vi "QueueMultiPakect_Snapshot.vi"(8 "no error":errorcluster, 11 "EndSession":bool=TRUE) -> (0 "error out":errorcluster={"status"=FALSE, "code"=1073676294, "source"="VISA Read in SerialCOM.vi->Queue MultiPakect-13.vi->getvideo.vi->Focus Routine.vi->Focus Routine.vi.ProxyCaller"}, 1 "success?":bool=TRUE, 2 "ImageData":u8[](array[numeric]) format="%x", 5 "RecvBuff":string, 6 "Done":bool=TRUE)   [LabVIEW 2014]
doc: "Demonstrates general use of Obtain Queue, queues and the effects different settings have on queue behavior. It uses a queue to pass data between an Enqueue loop (producing data) and a Dequeue loop (consuming data). If both loops run at the same speed, the queue does not fill up.\n\nWhen the Enqueue loop runs fast and the Dequeue loop runs slow, the queue quickly fills up and the Enqueue loop must wait for the Dequeue loop to remove elements. If the Enqueue loop runs slow and the Dequeue loop runs fast, the queue is quickly emptied and the Dequeue loop must wait for the Enqueue loop to insert elements."
panel:
  out "SendEndSession":bool
  out "max":u32
  out "Raw Data":u8[](array[numeric]) format="%x"
  out "Num_images":dbl=2.0
  out "readtime 2":u32=395
  out "RecvBuff 2":string
  out "#Ends":u32
  out "source":string="VISA Read in SerialCOM.vi->Queue MultiPakect-13.vi->getvideo.vi->Focus Routine.vi->Focus Routine.vi.ProxyCaller"
  out "Pakect":u8[](array[numeric])=[152, 180, 0, 0, 18, 18, 18, 18, 19, 18, 19, 18, 18, 19, 18, 19, 18, 18, 18, 18, 18, 19, 18, 18, 18, 18, 18, 18, 18, 18, 18, 18, 18, 18, 19, 18, 19, 18, 18, 18, 18, 18, 19, 18, 18, 18, 18, 18, 18, 18, 18, 18, 19, 19, 18, 18, 18, 18, 19, 19, 18, 19, 18, 18, 18, 18, 18, 18, 18, 18, 18, 18, 19, 18, 19, 18, 19, 18, 19, 18, 18, 18, 18, 19, 18, 19, 18, 18, 18, 19, 19, 18, 18, 18, 18, 18, 18, 18, 18, 18, 18, 19, 18, 18, 18, 18, 18, 18, 19, 18, 18, 18, 19, 18, 18, 18, 19, 19, 18, 18, 18, 18, 19, 19, 18, 18, 18, 19, 19, 18, 18, 18, 18, 19, 18, 18, 18, 18, 18, 18, 18, 18, 18, 19, 18, 18, 18, 19, 18, 18, 18, 18, 244, 43]
  out "End paks":bool=TRUE
  out "Index":u32=200346
  out "#Pakects":u32=783
  out "# in queue":i32
  out "readtime":u32=395
  out "DeEnque Loop":i32=879
  out "StartTime":u32=22222026
  out "Bytes At Port Loop":i32=1757
  out "Bytes at Port":u32
  out "Enque Loop":i32=391
  out "Bytes Read":u32=200346
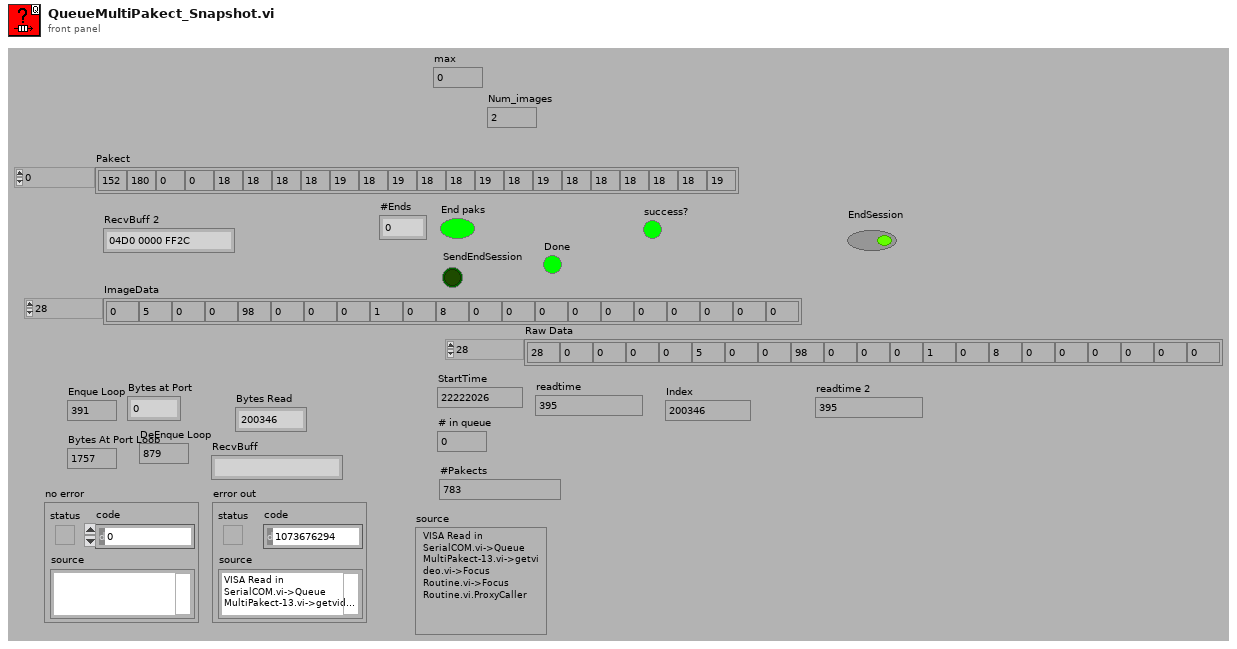
[diagram p1: front panel]
types:
  T1 = enum16{"OpenPort", "Initial Serial Port", "Write", "ByteRead", "Read", "ClearBuff", "Close"}
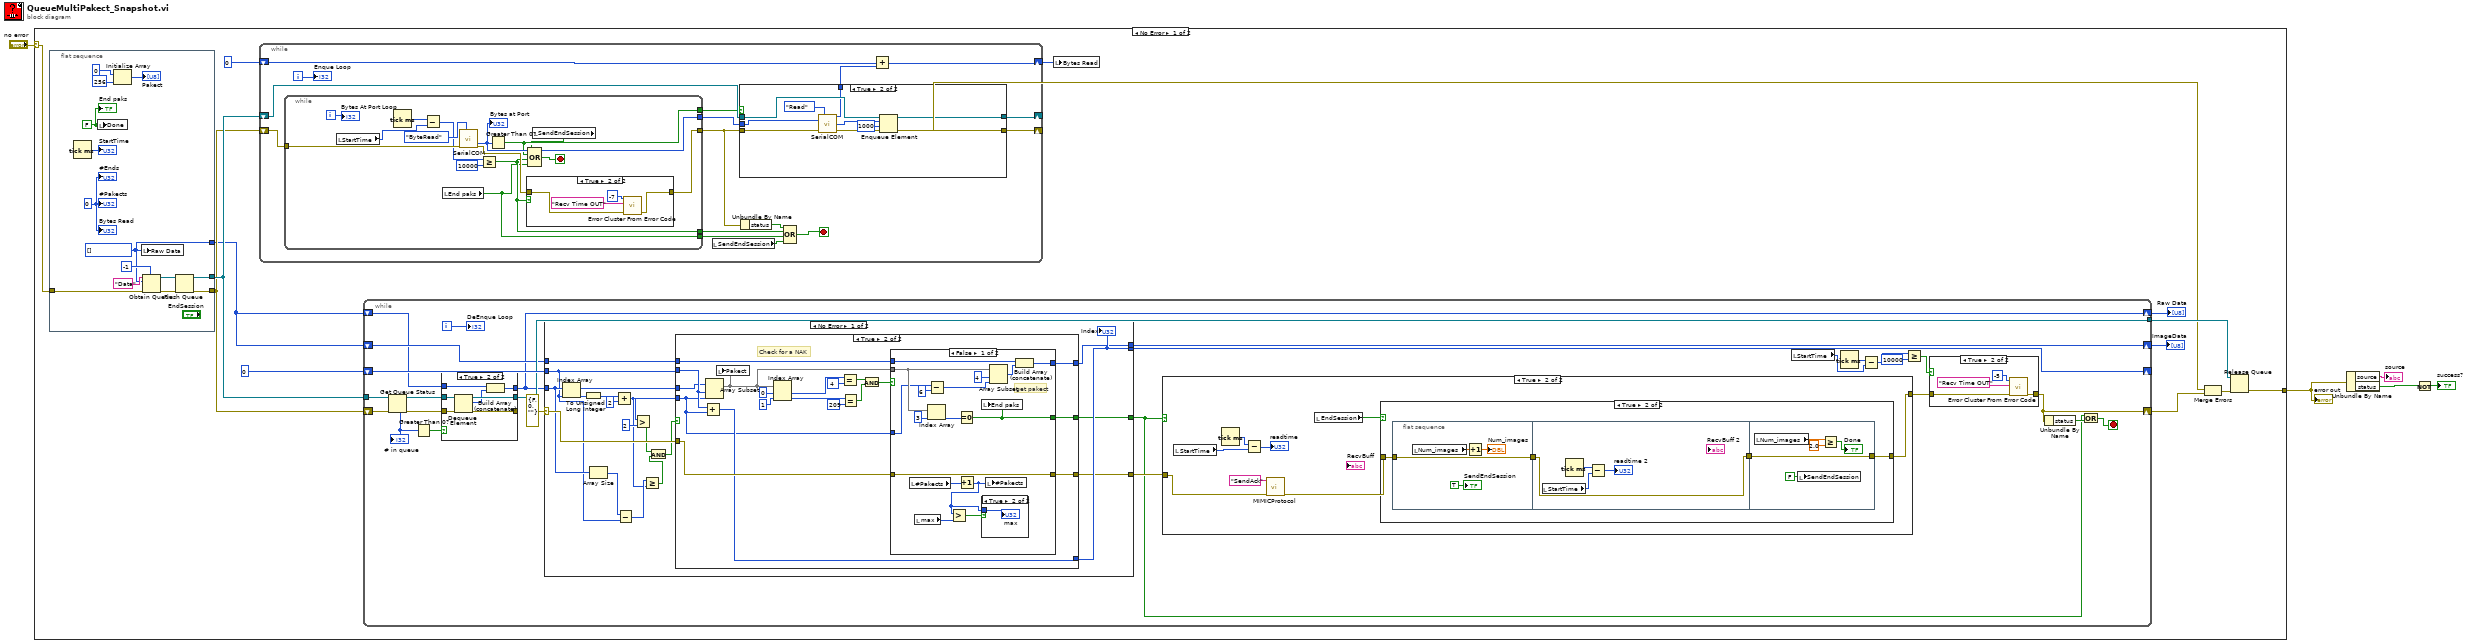
[diagram p0: block diagram]
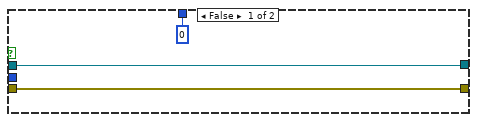
[diagram p3: hidden frame]
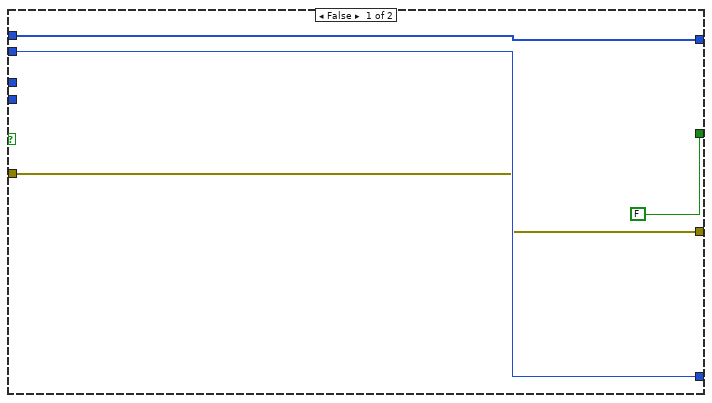
[diagram p4: hidden frame]
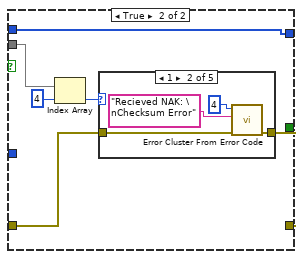
[diagram p6: hidden frame]
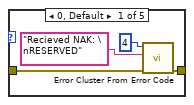
[diagram p7: hidden frame]
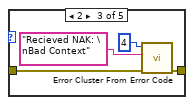
[diagram p8: hidden frame]
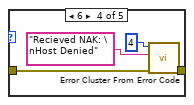
[diagram p9: hidden frame]
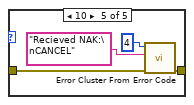
[diagram p10: hidden frame]
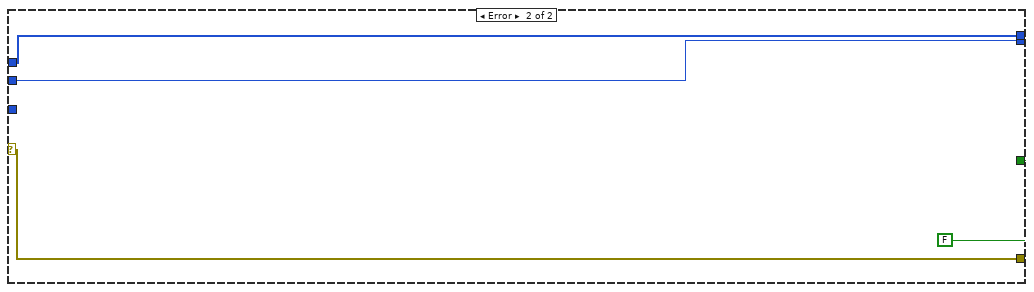
[diagram p11: hidden frame]
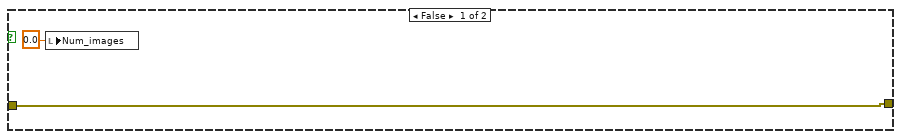
[diagram p15: hidden frame]
diagram:
  n1 = case shown="No Error" "no error" {
    selector: "no error" -> [w10 w240]
    tunnel: [w9 w240] -> w2
    frame No Error {
      n2 = flat-sequence {
        tunnel: [w29] -> w16
        tunnel: [w27] -> w8
        tunnel: [w26] -> w6
        tunnel: w10 -> [w21]
        frame #0 {
          w20 = u32 0 ("Bytes Read")
          w22 = FALSE ("full")
          w26 = u8[] []
          n3 = Tick Count (ms)() -> (millisecond timer value=→"StartTime":u32)
          n4 = local write "Done"(w22) -> ()
          n5 = Initialize Array(u8 0 ("element"), 256 ("dimension size")) -> (→"Pakect":u8[])
          n6 = local write "Raw Data"(w26) -> ()
          n7 = Obtain Queue(max queue size (-1, unlimited)=-1, name (unnamed)="Data", element data type=w26, error in (no error)=w21) -> (queue out=w30:refnum<queue>, error out=w28:errorcluster)  [unwired: 1 in, 1 out]
          n8 = Flush Queue(queue=w30, error in (no error)=w28) -> (queue out=w29:refnum<queue>, error out=w27:errorcluster)  [unwired: 1 out]
          "Bytes Read" <- w20
          "#Pakects" <- w20
          "End paks" <- w22
          "#Ends" <- w20
        }
      }
      n9 = while {
        shift-right: [w46] -> w19
        shift-left: u32 0 ("Bytes Read") -> [w48]
        shift-right: [w44] -> w13
        shift-left: w8 -> [w45]
        shift-right: [w38] -> _
        shift-left: w16 -> [w49]
        i -> [w42]
        stop <- w43 stop-if-true
        n10 = while {
          tunnel: [w54] -> w40
          tunnel: [w56] -> w47
          tunnel: w45 -> [w63]
          tunnel: [w53] -> w41
          tunnel: [w51] -> w39
          tunnel: [w52] -> w36
          i -> [w62]
          stop <- w57 stop-if-true
          n11 = local read "StartTime"() -> (w60:u32)
          n12 = Tick Count (ms)() -> (millisecond timer value=w61:u32)
          n13 = Subtract(x=w61, y=w60) -> (x-y=w59:u32)
          n14 = local read "End paks"() -> (w51:bool)
          n15 = call "SerialCOM.vi"("Function"=T1."ByteRead", "error in (no error)"=w63) -> ("Bytes at Port"=w56:u32, "error out"=w55:errorcluster)  [unwired: 8 in, 4 out]
          "Bytes at Port" <- w56
          n16 = Greater Or Equal?(x=w59, y=u32 10000) -> (x >= y?=w52:bool)
          n17 = Greater Than 0?(x=w56) -> (x > 0?=w53:bool)
          n18 = case shown="True" w52 {
            tunnel: w55 -> [w65 w69]
            tunnel: [w65 w68] -> w54
            frame False {
            }
            frame True {
              n19 = call <vilib>:"Error Cluster From Error Code.vi"("error in (no error)"=w69, "error message (\"\")"="Recv Time OUT" ("error message (\"\")"), "error code (0)"=-7) -> ("error out"=w68:errorcluster)  [unwired: 6 in]
            }
          }
          n20 = local read "SendEndSession"() -> (w50:bool)
          n21 = Compound Arithmetic op=OR(w50, w53, w52, w51) -> (w57:bool)
          "Bytes At Port Loop" <- w62
        }
        n22 = local read "SendEndSession"() -> (w34:bool)
        n23 = case shown="True" w41 {
          tunnel: w40 -> [w72 w79]
          tunnel: w47 -> [_ w77]
          tunnel: w49 -> [w71 w81]
          tunnel: [w72 w75] -> w44
          tunnel: [w71 w76] -> w38
          tunnel: [u32 0 ("return count") w78] -> w37
          frame False {
          }
          frame True {
            n24 = call "SerialCOM.vi"("Function"=T1."Read", "byte count"=w77, "error in (no error)"=w79) -> ("return count"=w78:u32, "array Out"=w74:u8[], "error out"=w80:errorcluster)  [unwired: 7 in, 3 out]
            n25 = Enqueue Element(queue=w81, element=w74, timeout in ms (-1)=1000, error in (no error)=w80) -> (queue out=w76:refnum<queue>, error out=w75:errorcluster)  [unwired: 1 out]
          }
        }
        n26 = Unbundle By Name(w40) -> ("status"=w35:bool)
        n27 = Compound Arithmetic op=OR(w35, w36, w39, w34) -> (w43:bool)
        n28 = Add(x=w48, y=w37) -> (x+y=w46:u32)
        "Enque Loop" <- w42
      }
      n29 = while {
        tunnel: w16 -> [w107]
        tunnel: [w102] -> w17
        shift-right: [w94] -> w12
        shift-left: w8 -> [w108]
        shift-right: [w101] -> _
        shift-left: u32 0 ("#Pakects") -> [w105]
        shift-right: [w92] -> w11
        shift-left: w6 -> [w93]
        shift-right: [w85] -> w7
        shift-left: w6 -> [w84]
        i -> [w106]
        stop <- w89 stop-if-true
        n30 = Get Queue Status(queue=w107, error in (no error)=w108) -> (queue out=w103:refnum<queue>, error out=w104:errorcluster, # elements in queue=w86:i32)  [unwired: 1 in, 5 out]
        "# in queue" <- w86
        n31 = Greater Than 0?(x=w86) -> (x > 0?=w87:bool)
        n32 = case shown="True" w87 {
          tunnel: w104 -> [w203 w206]
          tunnel: [w203 w205] -> _
          tunnel: w103 -> [w204 w211]
          tunnel: [w204 w210] -> w102
          tunnel: w84 -> [w202 w209]
          tunnel: [w202 w207] -> w85
          frame False {
          }
          frame True {
            n33 = Dequeue Element(queue=w211, error in (no error)=w206) -> (queue out=w210:refnum<queue>, element=w208:u8[], error out=w205:errorcluster)  [unwired: 2 out]
            n34 = Build Array (concatenate)(w209, w208) -> (w207:u8[])
          }
        }
        n35 = case shown="No Error" errorcluster {"status"=FALSE, "code"=0, "source"=""} ("error IO") {
          selector: errorcluster {"status"=FALSE, "code"=0, "source"=""} ("error IO") -> [w117 w196]
          tunnel: w105 -> [w109 w194]
          tunnel: [w123 w194] -> w101
          tunnel: [w122 w196] -> w100
          tunnel: w93 -> [w120 w195]
          tunnel: [w119 w195] -> w92
          tunnel: w85 -> [w116 _]
          tunnel: [w118 FALSE] -> w90
          frame No Error {
            n36 = Index Array(array=w116, index=w109) -> (element=w124:u8)
            n37 = To Unsigned Long Integer(number=w124) -> (unsigned 32bit integer=w125:u32)
            n38 = Array Size(array=w116) -> (size(s)=w115:i32)
            n39 = Add(x=w125, y=u32 2) -> (x+y=w110:u32)
            n40 = Subtract(x=w115, y=w109) -> (x-y=w111:u32)
            n41 = Greater?(x=w110, y=u32 2) -> (0:w114:bool)
            n42 = Greater Or Equal?(x=w111, y=w110) -> (x >= y?=w113:bool)
            n43 = And(x=w114, y=w113) -> (x .and. y?=w112:bool)
            n44 = case shown="True" w112 {
              tunnel: [w127 w143] -> w119
              tunnel: w109 -> [w129 w141]
              tunnel: w117 -> [w128 w140]
              tunnel: [w129 w136] -> w123
              tunnel: [w128 w135] -> w122
              tunnel: w116 -> [_ w134]
              tunnel: [FALSE w133] -> w118
              tunnel: w110 -> [_ w132]
              tunnel: w120 -> [w127 w131]
              frame False {
              }
              frame True {
                # "Check for a NAK"
                n45 = Add(x=w141, y=w132) -> (x+y=w136:u32)
                n46 = Array Subset(array=w134, index=w141, length=w132) -> (w137:u8[])
                n47 = local write "Pakect"(w137) -> ()
                n48 = Index Array(array=w137, index #1=0 ("index"), index #2=1 ("index")) -> (element #1=w149:u8, element #2=w138:u8)
                n49 = Equal?(x=w149, y=u8 4) -> (x = y?=w145:bool)
                n50 = Equal?(x=w138, y=u8 209) -> (x = y?=w146:bool)
                n51 = Compound Arithmetic op=AND(w145, w146) -> (w142:bool)
                n52 = case shown="False" w142 {
                  tunnel: [w156 w167] -> w143
                  tunnel: w137 -> [w160 w170]
                  tunnel: w132 -> [w159 _]
                  tunnel: w140 -> [w162 w172]
                  tunnel: [w162 w168] -> w135
                  tunnel: [w154 _] -> w133
                  tunnel: w131 -> [w155 w167]
                  frame False {
                    # "get pakect"
                    n53 = local read "#Pakects"() -> (w153:u32)
                    n54 = local read "max"() -> (w150:u32)
                    n55 = Subtract(x=w159, y=u32 6) -> (x-y=w163:u32)
                    n56 = Index Array(array=w160, index=3) -> (element=w158:u8)
                    n57 = Equal To 0?(x=w158) -> (x = 0?=w154:bool)
                    n58 = Increment(x=w153) -> (x+1=w151:u32)
                    n59 = Greater?(x=w151, y=w150) -> (0:w152:bool)
                    n60 = local write "End paks"(w154) -> ()
                    n61 = case shown="True" w152 {
                      tunnel: w151 -> [_ w166]
                      frame False {
                      }
                      frame True {
                        "max" <- w166
                      }
                    }
                    n62 = local write "#Pakects"(w151) -> ()
                    n63 = Array Subset(array=w160, index=4, length=w163) -> (w157:u8[])
                    n64 = Build Array (concatenate)(w155, w157) -> (w156:u8[])
                  }
                  frame True {
                    n65 = Index Array(array=w170, index=4) -> (element=w169:u8)
                    n66 = case shown="1" w169 {
                      tunnel: w172 -> [w176 w180 w184 w188 w192]
                      tunnel: [w175 w179 w183 w187 w191] -> w168
                      frame 0, Default {
                        n67 = call <vilib>:"Error Cluster From Error Code.vi"("error in (no error)"=w176, "error message (\"\")"="Recieved NAK: \nRESERVED" ("error message (\"\")"), "error code (0)"=4) -> ("error out"=w175:errorcluster)  [unwired: 6 in]
                      }
                      frame 1 {
                        n68 = call <vilib>:"Error Cluster From Error Code.vi"("error in (no error)"=w180, "error message (\"\")"="Recieved NAK: \nChecksum Error" ("error message (\"\")"), "error code (0)"=4) -> ("error out"=w179:errorcluster)  [unwired: 6 in]
                      }
                      frame 2 {
                        n69 = call <vilib>:"Error Cluster From Error Code.vi"("error in (no error)"=w184, "error message (\"\")"="Recieved NAK: \nBad Context" ("error message (\"\")"), "error code (0)"=4) -> ("error out"=w183:errorcluster)  [unwired: 6 in]
                      }
                      frame 6 {
                        n70 = call <vilib>:"Error Cluster From Error Code.vi"("error in (no error)"=w188, "error message (\"\")"="Recieved NAK: \nHost Denied" ("error message (\"\")"), "error code (0)"=4) -> ("error out"=w187:errorcluster)  [unwired: 6 in]
                      }
                      frame 10 {
                        n71 = call <vilib>:"Error Cluster From Error Code.vi"("error in (no error)"=w192, "error message (\"\")"="Recieved NAK:\nCANCEL" ("error message (\"\")"), "error code (0)"=4) -> ("error out"=w191:errorcluster)  [unwired: 6 in]
                      }
                    }
                  }
                }
              }
            }
            "Index" <- w123
          }
          frame Error {
          }
        }
        n72 = case shown="True" w90 {
          tunnel: w100 -> [w212 w215]
          tunnel: [w212 w216] -> w88
          frame False {
          }
          frame True {
            n73 = local read "StartTime"() -> (w218:u32)
            n74 = Tick Count (ms)() -> (millisecond timer value=w219:u32)
            n75 = Subtract(x=w219, y=w218) -> (x-y=→"readtime":u32)
            n76 = call "MIMICProtocol.vi"("Error In"=w215, "MIMIC_Command"="SendAck") -> ("Error Out"=w214:errorcluster)  [unwired: 3 in, 3 out]
            n77 = local read "EndSession"() -> (w217:bool)
            n78 = case shown="True" w217 {
              tunnel: w214 -> [w222 w225]
              tunnel: [w222 w223] -> w216
              frame False {
                n79 = local write "Num_images"(0.0 ("Num_images")) -> ()
              }
              frame True {
                n80 = flat-sequence {
                  tunnel: [w228] -> w226
                  tunnel: w225 -> [w228]
                  tunnel: w226 -> [w231]
                  tunnel: [w231] -> w224
                  tunnel: w224 -> [w236]
                  tunnel: [w236] -> w223
                  frame #0 {
                    n81 = local read "Num_images"() -> (w229:dbl)
                    n82 = Increment(x=w229) -> (x+1=→"Num_images":dbl)
                    "SendEndSession" <- TRUE ("SendEndSession")
                  }
                  frame #1 {
                    n83 = local read "StartTime"() -> (w234:u32)
                    n84 = Tick Count (ms)() -> (millisecond timer value=w233:u32)
                    n85 = Subtract(x=w233, y=w234) -> (x-y=→"readtime 2":u32)
                  }
                  frame #2 {
                    n86 = local read "Num_images"() -> (w237:dbl)
                    n87 = local write "SendEndSession"(FALSE ("SendEndSession")) -> ()
                    n88 = Greater Or Equal?(x=w237, y=2.0) -> (x >= y?=→"Done":bool)
                  }
                }
              }
            }
          }
        }
        n89 = local read "StartTime"() -> (w96:u32)
        n90 = Tick Count (ms)() -> (millisecond timer value=w97:u32)
        n91 = Subtract(x=w97, y=w96) -> (x-y=w98:u32)
        n92 = Greater Or Equal?(x=w98, y=u32 10000) -> (x >= y?=w95:bool)
        n93 = case shown="True" w95 {
          tunnel: w88 -> [w197 w201]
          tunnel: [w197 w200] -> w94
          frame False {
          }
          frame True {
            n94 = call <vilib>:"Error Cluster From Error Code.vi"("error in (no error)"=w201, "error message (\"\")"="Recv Time OUT" ("error message (\"\")"), "error code (0)"=-5) -> ("error out"=w200:errorcluster)  [unwired: 6 in]
          }
        }
        n95 = Unbundle By Name(w94) -> ("status"=w91:bool)
        n96 = Compound Arithmetic op=OR(w90, w91) -> (w89:bool)
        "DeEnque Loop" <- w106
      }
      "ImageData" <- w11
      "Raw Data" <- w7
      n97 = local write "Bytes Read"(w19) -> ()
      n98 = Merge Errors(w13, w12) -> (w18:errorcluster)
      n99 = Release Queue(queue=w17, error in (no error)=w18) -> (error out=w9:errorcluster)  [unwired: 3 out]
    }
    frame Error {
    }
  }
  "error out" <- w2
  n100 = Unbundle By Name(w2) -> ("source"=→"source":string, "status"=w4:bool)
  n101 = Not(x=w4) -> (.not. x?=→"success?":bool)
